vi "StateShooter2.vi"(1 "Master State":enum16{"Normal", "Climb"}(ring)) -> (0 "Shooter Firing":bool)   [LabVIEW 2020]
doc: "Performs all of the calculations and decisions related to the shooter including the cowl positon."
uses:
  a6f50b4d-1f67-4415-9d76-8f68db1e14ec.vi
  drivercommands.vi
  robotoutputs.vi
  robotconstants.vi
  driverdata.vi
  autonomousinfo.vi
  sensordata.vi
panel:
  in  "Acceptable Upper Shooter Error (rpm)":dbl=250.0
  in  "Minimum Range (in)":dbl=50.0
  in  "Maximum Range (in)":dbl=300.0
  in  "Max Robot Ground Speed (ft/s)":dbl=7.0
  in  "Acceptable Cowl Error (deg)":dbl=2.0
  in  "Acceptable Lower Shooter Error (rpm)":dbl=150.0
  in  "Settling Time (ms)":u32=100
  in  "Shooter Prespin (ms)":u32=5000
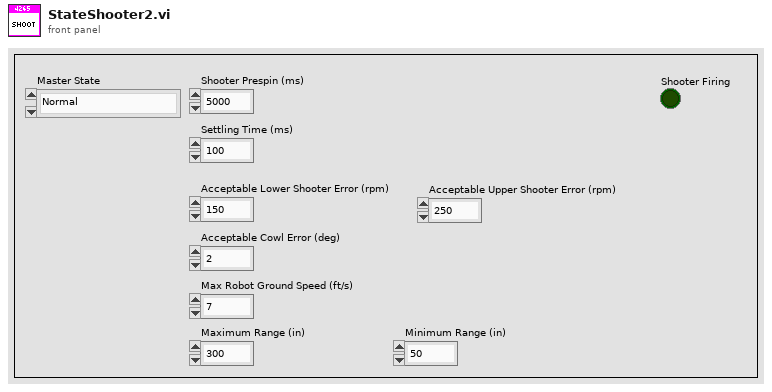
[diagram p1: front panel]
types:
  T1 = enum16{"Targetting Computer", "Position 1", "Position 2", "Position 3", "Position 4"}
  T2 = typedef "WPI_DriverStationAllianceInfo.ctl" = enum16{"Red", "Blue", "Invalid"}
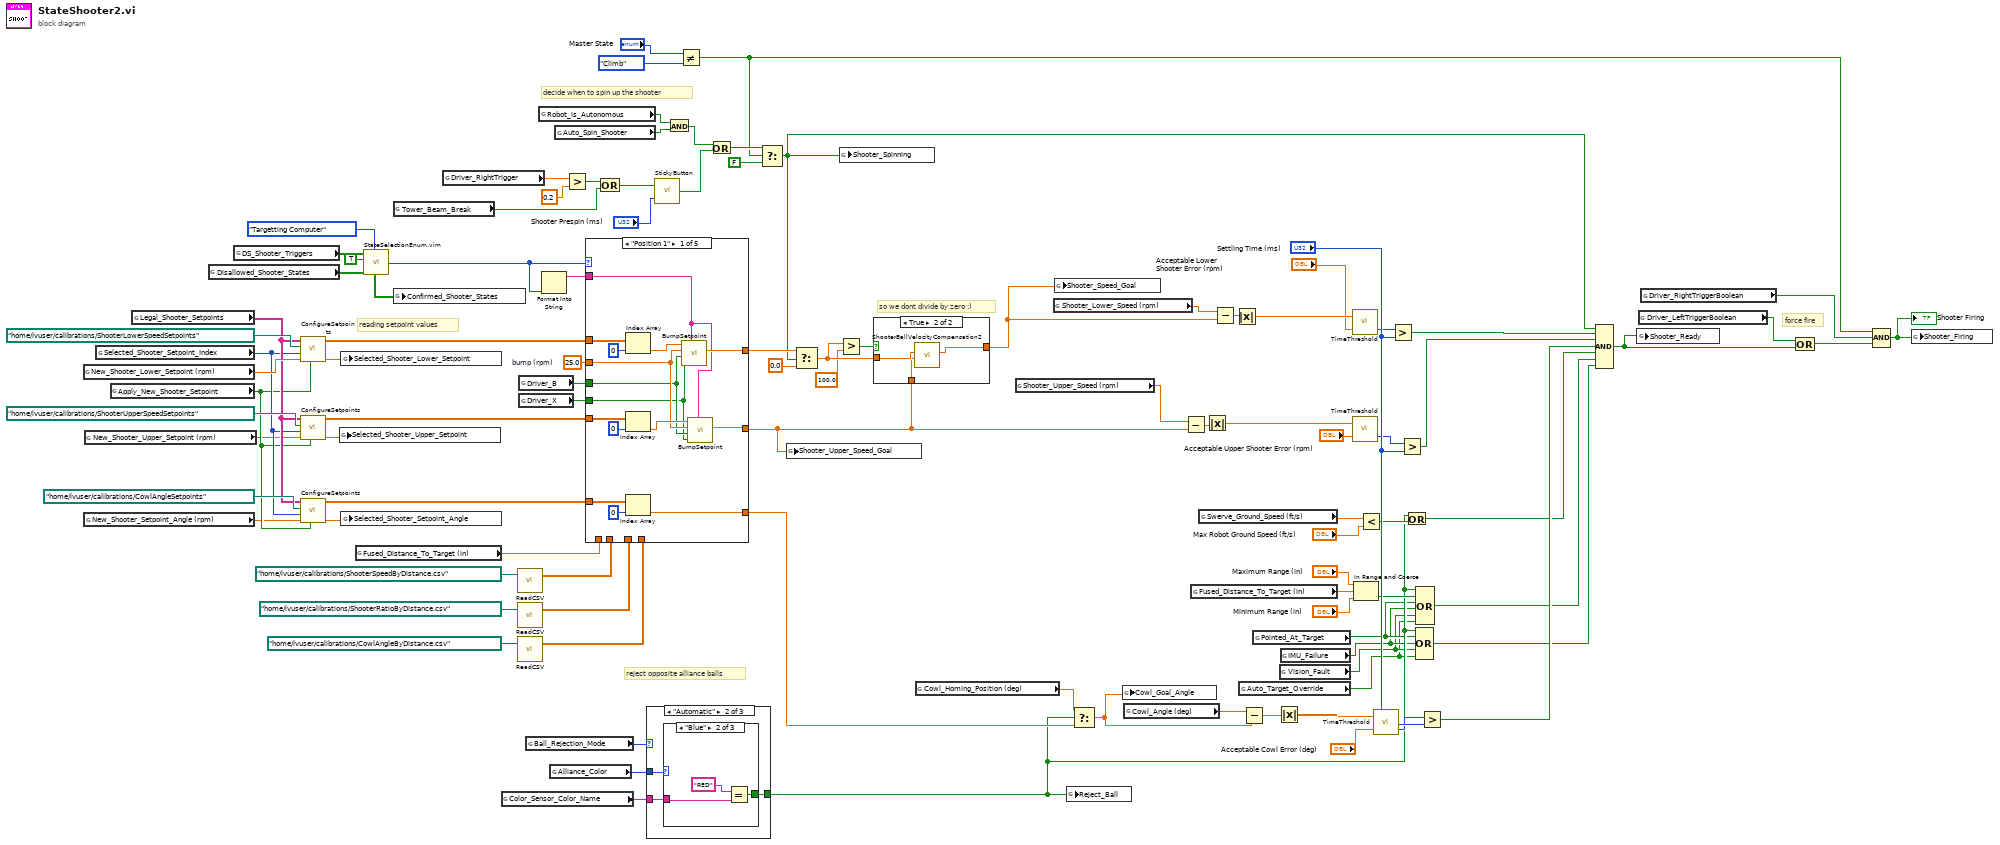
[diagram p0: block diagram]
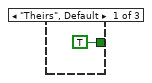
[diagram p3: hidden frame]
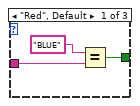
[diagram p4: hidden frame]
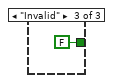
[diagram p5: hidden frame]
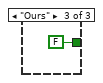
[diagram p6: hidden frame]
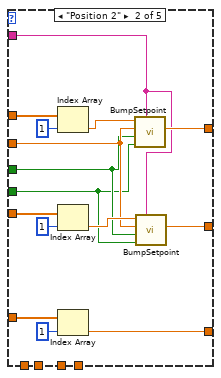
[diagram p7: hidden frame]
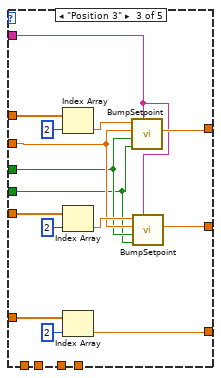
[diagram p8: hidden frame]
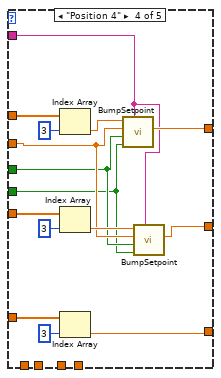
[diagram p9: hidden frame]
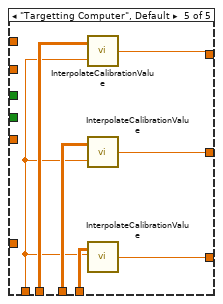
[diagram p10: hidden frame]
diagram:
  w48 = 25.0  # bump (rpm)
  # "so we dont divide by zero :)"
  # "reject opposite alliance balls"
  # "force fire"
  # "reading setpoint values"
  # "decide when to spin up the shooter"
  n1 = global read "driverdata.vi" "New_Shooter_Lower_Setpoint (rpm)"() -> (w94:dbl)
  n2 = global read "driverdata.vi" "New_Shooter_Setpoint_Angle (rpm)"() -> (w84:dbl)
  n3 = global read "driverdata.vi" "New_Shooter_Upper_Setpoint (rpm)"() -> (w85:dbl)
  n4 = global read "driverdata.vi" "Selected_Shooter_Setpoint_Index"() -> (w88:i32)
  n5 = global read "driverdata.vi" "Apply_New_Shooter_Setpoint"() -> (w86:bool)
  n6 = global read "robotconstants.vi" "Legal_Shooter_Setpoints"() -> (w89:string[])
  n7 = global read "robotoutputs.vi" "Disallowed_Shooter_States"() -> (w98:bool[])
  n8 = global read "drivercommands.vi" "DS_Shooter_Triggers"() -> (w100:bool[])
  n9 = call "ConfigureSetpoints.vi"("Apply New Setpoint"=w86, "New Setpoint"=w94, "Selected Setpoint Index"=w88, "Setpoint Save Location"=path "/home/lvuser/calibrations/ShooterLowerSpeedSetpoints", "Setpoint Names"=w89) -> ("Selected Setpoint Value"=w83:dbl, "Setpoints"=w93:dbl[])  [unwired: 5 in]
  n10 = call "ConfigureSetpoints.vi"("Apply New Setpoint"=w86, "New Setpoint"=w85, "Selected Setpoint Index"=w88, "Setpoint Save Location"=path "/home/lvuser/calibrations/ShooterUpperSpeedSetpoints", "Setpoint Names"=w89) -> ("Selected Setpoint Value"=w82:dbl, "Setpoints"=w91:dbl[])  [unwired: 5 in]
  n11 = call "ConfigureSetpoints.vi"("Apply New Setpoint"=w86, "New Setpoint"=w84, "Selected Setpoint Index"=w88, "Setpoint Save Location"=path "/home/lvuser/calibrations/CowlAngleSetpoints", "Setpoint Names"=w89) -> ("Selected Setpoint Value"=w81:dbl, "Setpoints"=w87:dbl[])  [unwired: 5 in]
  n12 = global write "robotoutputs.vi" "Selected_Shooter_Upper_Setpoint"(w82) -> ()
  n13 = global write "robotoutputs.vi" "Selected_Shooter_Lower_Setpoint"(w83) -> ()
  n14 = global write "robotoutputs.vi" "Selected_Shooter_Setpoint_Angle"(w81) -> ()
  n15 = global read "sensordata.vi" "Fused_Distance_To_Target (in)"() -> (w51:dbl)
  n16 = call "StateSelectionEnum.vim"("Enum Def"=T1."Targetting Computer", "Disallowed States"=w98, "Enable Edge Trigger"=TRUE, "State Triggers"=w100) -> ("Selected State"=w45:T1, "Confirmed States"=w97:bool[])  [unwired: 1 in]
  n17 = global read "sensordata.vi" "Tower_Beam_Break"() -> (w3:bool)
  n18 = global write "robotoutputs.vi" "Confirmed_Shooter_States"(w97) -> ()
  n19 = global read "drivercommands.vi" "Driver_RightTrigger"() -> (w78:dbl)
  n20 = global read "sensordata.vi" "Color_Sensor_Color_Name"() -> (w24:string)
  n21 = call "ReadCSV.vi"("File Path (.csv)"=path "/home/lvuser/calibrations/ShooterSpeedByDistance.csv" ("Setpoint Save Location")) -> ("Data (index by row)"=w52:dbl[][])  [unwired: 1 in, 1 out]
  n22 = call "ReadCSV.vi"("File Path (.csv)"=path "/home/lvuser/calibrations/ShooterRatioByDistance.csv" ("Setpoint Save Location")) -> ("Data (index by row)"=w50:dbl[][])  [unwired: 1 in, 1 out]
  n23 = call "ReadCSV.vi"("File Path (.csv)"=path "/home/lvuser/calibrations/CowlAngleByDistance.csv" ("Setpoint Save Location")) -> ("Data (index by row)"=w49:dbl[][])  [unwired: 1 in, 1 out]
  n24 = global read "drivercommands.vi" "Driver_B"() -> (w47:bool)
  n25 = global read "drivercommands.vi" "Driver_X"() -> (w46:bool)
  n26 = global read "driverdata.vi" "Ball_Rejection_Mode"() -> (w21:enum16{"Theirs", "Automatic", "Ours"})
  n27 = global read "driverdata.vi" "Robot_is_Autonomous"() -> (w71:bool)
  n28 = Format Into String(w45) -> (resulting string=w44:string)  [unwired: 3 in, 1 out]
  n29 = global read "driverdata.vi" "Alliance_Color"() -> (w25:T2)
  n30 = global read "autonomousinfo.vi" "Auto_Spin_Shooter"() -> (w72:bool)
  n31 = Greater?(x=w78, y=0.2) -> (0:w76:bool)
  n32 = case shown="\"Position 1\"" w45 {
    tunnel: w93 -> [w115 w127 w142 w157 _]
    tunnel: w91 -> [w112 w126 w141 w156 _]
    tunnel: w87 -> [w110 w125 w140 w155 _]
    tunnel: [w107 w122 w137 w153 w166] -> w80
    tunnel: [w106 w121 w136 w147 w164] -> w1
    tunnel: [w109 w124 w139 w154 w161] -> w23
    tunnel: w52 -> [_ _ _ _ w167]
    tunnel: w51 -> [_ _ _ _ w162]
    tunnel: w50 -> [_ _ _ _ w165]
    tunnel: w49 -> [_ _ _ _ w163]
    tunnel: w48 -> [w103 w119 w134 w150 _]
    tunnel: w47 -> [w102 w118 w133 w149 _]
    tunnel: w46 -> [w101 w117 w132 w148 _]
    tunnel: w44 -> [w105 w116 w131 w146 _]
    frame "Position 1" {
      n33 = Index Array(array=w115, index=0) -> (element=w108:dbl)
      n34 = Index Array(array=w112, index=0) -> (element=w104:dbl)
      n35 = Index Array(array=w110, index=0) -> (element=w109:dbl)
      n36 = call "BumpSetpoint.vi"("Setpoint Name"=w105, "Bump Down Trigger"=w101, "Bump Up Trigger"=w102, "Bump Increment"=w103, "Original Setpoint"=w108) -> ("Bumped Setpoint"=w107:dbl)  [unwired: 6 in]
      n37 = call "BumpSetpoint.vi"("Setpoint Name"=w105, "Bump Down Trigger"=w101, "Bump Up Trigger"=w102, "Bump Increment"=w103, "Original Setpoint"=w104) -> ("Bumped Setpoint"=w106:dbl)  [unwired: 6 in]
    }
    frame "Position 2" {
      n38 = Index Array(array=w127, index=1) -> (element=w123:dbl)
      n39 = Index Array(array=w126, index=1) -> (element=w120:dbl)
      n40 = Index Array(array=w125, index=1) -> (element=w124:dbl)
      n41 = call "BumpSetpoint.vi"("Setpoint Name"=w116, "Bump Down Trigger"=w117, "Bump Up Trigger"=w118, "Bump Increment"=w119, "Original Setpoint"=w123) -> ("Bumped Setpoint"=w122:dbl)  [unwired: 6 in]
      n42 = call "BumpSetpoint.vi"("Setpoint Name"=w116, "Bump Down Trigger"=w117, "Bump Up Trigger"=w118, "Bump Increment"=w119, "Original Setpoint"=w120) -> ("Bumped Setpoint"=w121:dbl)  [unwired: 6 in]
    }
    frame "Position 3" {
      n43 = Index Array(array=w142, index=2) -> (element=w138:dbl)
      n44 = Index Array(array=w141, index=2) -> (element=w135:dbl)
      n45 = Index Array(array=w140, index=2) -> (element=w139:dbl)
      n46 = call "BumpSetpoint.vi"("Setpoint Name"=w131, "Bump Down Trigger"=w132, "Bump Up Trigger"=w133, "Bump Increment"=w134, "Original Setpoint"=w138) -> ("Bumped Setpoint"=w137:dbl)  [unwired: 6 in]
      n47 = call "BumpSetpoint.vi"("Setpoint Name"=w131, "Bump Down Trigger"=w132, "Bump Up Trigger"=w133, "Bump Increment"=w134, "Original Setpoint"=w135) -> ("Bumped Setpoint"=w136:dbl)  [unwired: 6 in]
    }
    frame "Position 4" {
      n48 = Index Array(array=w157, index=3) -> (element=w152:dbl)
      n49 = Index Array(array=w156, index=3) -> (element=w151:dbl)
      n50 = Index Array(array=w155, index=3) -> (element=w154:dbl)
      n51 = call "BumpSetpoint.vi"("Setpoint Name"=w146, "Bump Down Trigger"=w148, "Bump Up Trigger"=w149, "Bump Increment"=w150, "Original Setpoint"=w152) -> ("Bumped Setpoint"=w153:dbl)  [unwired: 6 in]
      n52 = call "BumpSetpoint.vi"("Setpoint Name"=w146, "Bump Down Trigger"=w148, "Bump Up Trigger"=w149, "Bump Increment"=w150, "Original Setpoint"=w151) -> ("Bumped Setpoint"=w147:dbl)  [unwired: 6 in]
    }
    frame "Targetting Computer", Default {
      n53 = call "InterpolateCalibrationValue.vi"("Input"=w162, "Calibration Data"=w167) -> ("Interpolated Output"=w166:dbl)
      n54 = call "InterpolateCalibrationValue.vi"("Input"=w162, "Calibration Data"=w165) -> ("Interpolated Output"=w164:dbl)
      n55 = call "InterpolateCalibrationValue.vi"("Input"=w162, "Calibration Data"=w163) -> ("Interpolated Output"=w161:dbl)
    }
  }
  n56 = Compound Arithmetic op=OR(w76, w3) -> (w75:bool)
  n57 = case shown="\"Automatic\"" w21 {
    tunnel: w25 -> [_ w171 _]
    tunnel: w24 -> [_ w170 _]
    tunnel: [TRUE w169 FALSE] -> w14
    frame "Theirs", Default {
    }
    frame "Automatic" {
      n58 = case shown="\"Blue\"" w171 {
        tunnel: w170 -> [w174 w176 _]
        tunnel: [w172 w175 FALSE] -> w169
        frame "Red", Default {
          n59 = Equal?(x="BLUE", y=w174) -> (x = y?=w172:bool)
        }
        frame "Blue" {
          n60 = Equal?(x="RED", y=w176) -> (x = y?=w175:bool)
        }
        frame "Invalid" {
        }
      }
    }
    frame "Ours" {
    }
  }
  n61 = call "StickyButton.vi"("Time threshold (ms)"="Shooter Prespin (ms)", "Button Input"=w75) -> ("Sticky Button"=w69:bool)
  n62 = And(x=w71, y=w72) -> (x .and. y?=w70:bool)
  n63 = Not Equal?(x="Master State", y=enum16{"Normal", "Climb"}."Climb" ("Master State")) -> (x != y?=w57:bool)
  n64 = Or(x=w70, y=w69) -> (x .or. y?=w68:bool)
  n65 = Select(t=w68, s=w57, f=FALSE) -> (s? t:f=w26:bool)
  n66 = global write "robotoutputs.vi" "Shooter_Upper_Speed_Goal"(w1) -> ()
  n67 = Select(t=w80, s=w26, f=0.0) -> (s? t:f=w10:dbl)
  n68 = Greater?(x=w10, y=100.0) -> (0:w8:bool)
  n69 = global write "robotoutputs.vi" "Shooter_Spinning"(w26) -> ()
  n70 = case shown="True" w8 {
    tunnel: w1 -> [_ w182]
    tunnel: w10 -> [w180 w183]
    tunnel: [w180 w181] -> w11
    frame False {
    }
    frame True {
      n71 = call "ShooterBallVelocityCompensation2.vi"("Shooter Upper Speed Goal"=w182, "Shooter Lower Speed Goal"=w183) -> ("Compensated Speed Goal"=w181:dbl)  [unwired: 9 in]
    }
  }
  n72 = global read "robotconstants.vi" "Cowl_Homing_Position (deg)"() -> (w19:dbl)
  n73 = global read "sensordata.vi" "Shooter_Upper_Speed (rpm)"() -> (w2:dbl)
  n74 = global read "sensordata.vi" "Shooter_Lower_Speed (rpm)"() -> (w43:dbl)
  n75 = global write "robotoutputs.vi" "Shooter_Speed_Goal"(w11) -> ()
  n76 = global write "robotoutputs.vi" "Reject_Ball"(w14) -> ()
  n77 = Select(t=w19, s=w14, f=w23) -> (s? t:f=w22:dbl)
  n78 = global write "robotoutputs.vi" "Cowl_Goal_Angle"(w22) -> ()
  n79 = global read "sensordata.vi" "Cowl_Angle (deg)"() -> (w37:dbl)
  n80 = Subtract(x=w2, y=w1) -> (x-y=w65:dbl)
  n81 = global read "sensordata.vi" "Fused_Distance_To_Target (in)"() -> (w29:dbl)
  n82 = global read "sensordata.vi" "Swerve_Ground_Speed (ft/s)"() -> (w31:dbl)
  n83 = Absolute Value(x=w65) -> (abs(x)=w41:dbl)
  n84 = Subtract(x=w43, y=w11) -> (x-y=w66:dbl)
  n85 = Absolute Value(x=w66) -> (abs(x)=w42:dbl)
  n86 = global read "driverdata.vi" "Auto_Target_Override"() -> (w4:bool)
  n87 = Subtract(x=w37, y=w22) -> (x-y=w64:dbl)
  n88 = global read "sensordata.vi" "Pointed_At_Target"() -> (w7:bool)
  n89 = Absolute Value(x=w64) -> (abs(x)=w61:dbl)
  n90 = global read "sensordata.vi" "Vision_Fault"() -> (w5:bool)
  n91 = global read "sensordata.vi" "IMU_Failure"() -> (w6:bool)
  n92 = call "TimeThreshold.vi"("Threshold"="Acceptable Lower Shooter Error (rpm)", "Current Value"=w42) -> ("Time Below Threshold (ms)"=w39:u32)  [unwired: 1 out]
  n93 = call "TimeThreshold.vi"("Threshold"="Acceptable Upper Shooter Error (rpm)", "Current Value"=w41) -> ("Time Below Threshold (ms)"=w38:u32)  [unwired: 1 out]
  n94 = In Range and Coerce(upper limit="Maximum Range (in)", x=w29, lower limit="Minimum Range (in)") -> (In Range?=w16:bool)  [unwired: 1 out]
  n95 = Less?(x=w31, y="Max Robot Ground Speed (ft/s)") -> (x < y?=w17:bool)
  n96 = call "TimeThreshold.vi"("Threshold"="Acceptable Cowl Error (deg)", "Current Value"=w61) -> ("Time Below Threshold (ms)"=w20:u32)  [unwired: 1 out]
  n97 = Greater?(x=w39, y="Settling Time (ms)") -> (0:w63:bool)
  n98 = Greater?(x=w38, y="Settling Time (ms)") -> (0:w62:bool)
  n99 = Or(x=w14, y=w17) -> (x .or. y?=w18:bool)
  n100 = Compound Arithmetic op=OR(w14, w7, w6, w5, w4) -> (w13:bool)
  n101 = Compound Arithmetic op=OR(w14, w16, w7, w6, w5, w4) -> (w15:bool)
  n102 = Greater?(x=w20, y="Settling Time (ms)") -> (0:w59:bool)
  n103 = Compound Arithmetic op=AND(w26, w63, w62, w59, w18, w15, w13) -> (w35:bool)
  n104 = global write "robotoutputs.vi" "Shooter_Ready"(w35) -> ()
  n105 = global read "drivercommands.vi" "Driver_LeftTriggerBoolean"() -> (w34:bool)
  n106 = global read "drivercommands.vi" "Driver_RightTriggerBoolean"() -> (w33:bool)
  n107 = Compound Arithmetic op=OR(w34, w35) -> (w32:bool)
  n108 = Compound Arithmetic op=AND(w57, w33, w32) -> (w56:bool)
  "Shooter Firing" <- w56
  n109 = global write "robotoutputs.vi" "Shooter_Firing"(w56) -> ()
